vi "HTML Video Steams.vi"(7 "Cameras 2":refnum<vi>, 8 "Exit":refnum<vi>, 10 "Video Feed 2":refnum<vi>, 11 "Automation Refnum in":refnum<k7>) -> (0 "error out":errorcluster, 3 "Automation Refnum out":refnum<k7>)   [LabVIEW 2017]
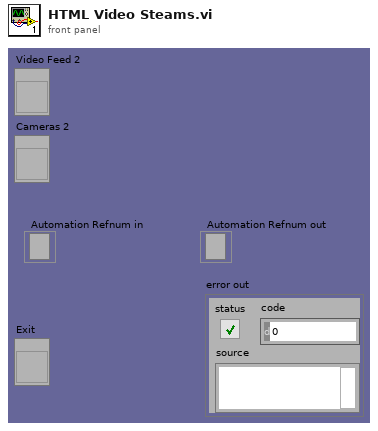
[diagram p1: front panel]
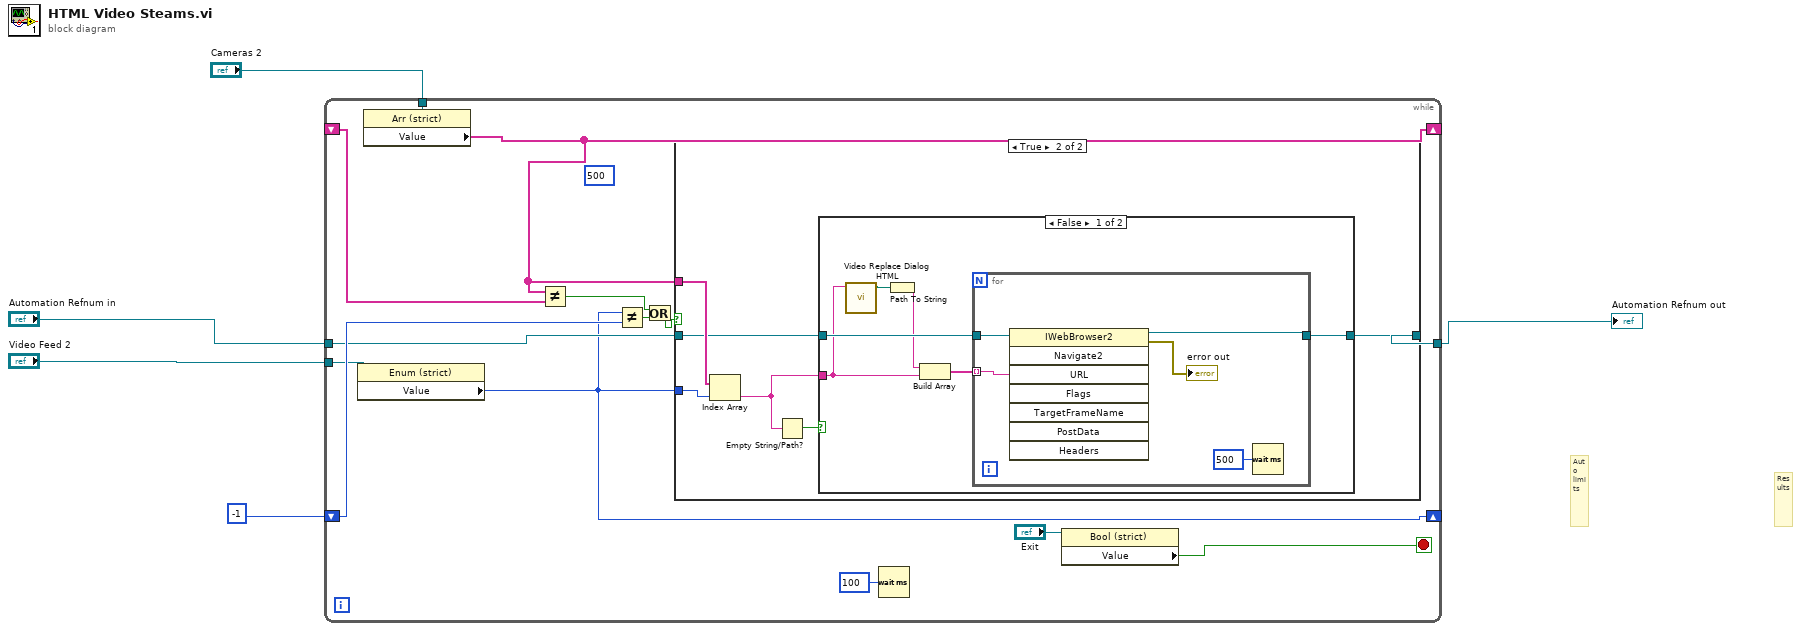
[diagram p0: block diagram]
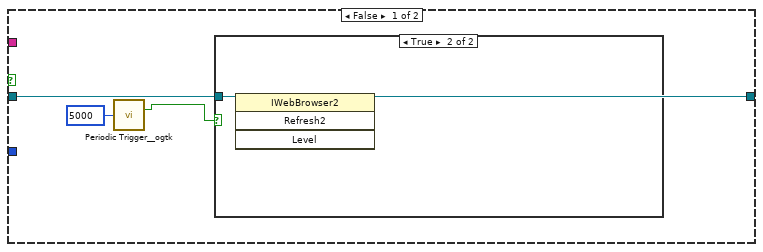
[diagram p2: hidden frame]
diagram:
  # "Results"
  # "Auto limits"
  n1 = while {
    shift-right: [w13] -> _
    shift-left: -1 -> [w18]
    tunnel: "Video Feed 2" -> [w14]
    tunnel: "Automation Refnum in" -> [w17]
    tunnel: [w19] -> w5
    shift-right: [w6] -> _
    shift-left: _ -> [w9]
    tunnel: "Cameras 2" -> [w7]
    stop <- w15 stop-if-true
    (unwired) 500
    n2 = property class="Enum (strict)"(reference=w14) -> ("Value"=w13:enum16{"Camera 1", "Camera2", "Mobile"})  [unwired: 1 in, 2 out]
    n3 = property class="Arr (strict)"(reference=w7) -> ("Value"=w6:string[])  [unwired: 1 in, 2 out]
    n4 = Not Equal?(x=w6, y=w9) -> (x != y?=w8:bool)
    n5 = Not Equal?(x=w13, y=w18) -> (x != y?=w11:bool)
    n6 = Or(x=w8, y=w11) -> (x .or. y?=w10:bool)
    n7 = case shown="True" w10 {
      tunnel: [w22 w29] -> w19
      tunnel: w6 -> [_ w28]
      tunnel: w13 -> [_ w27]
      tunnel: w17 -> [w22 w26]
      frame False {
        n8 = call <userlib>:"Periodic Trigger__ogtk.vi"("time (ms)"=u32 5000) -> ("Triggered"=w21:bool)  [unwired: 12 in, 2 out]
        n9 = case shown="True" w21 {
          tunnel: w22 -> [_ w23]
          frame False {
          }
          frame True {
            n10 = invoke class="IWebBrowser2" method="Refresh2"(reference=w23) -> ()  [unwired: 3 in, 4 out]
          }
        }
      }
      frame True {
        n11 = Index Array(array=w28, index=w27) -> (element=w25:string)
        n12 = Empty String/Path?(string/path=w25) -> (empty?=w24:bool)
        n13 = case shown="False" w24 {
          tunnel: [w35 w41] -> w29
          tunnel: w26 -> [w34 w41]
          tunnel: w25 -> [w31 _]
          frame False {
            n14 = call "Video Replace Dialog HTML.vi"("String"=w31) -> ("appended path"=w30:path)  [unwired: 10 in]
            n15 = Path To String(path=w30) -> (string=w33:string)
            n16 = Build Array(w33, w31) -> (w32:string[])
            n17 = for {
              tunnel: w32 -> [w37] mode=indexing
              tunnel: w34 -> [w38]
              tunnel: [w40] -> w35
              n18 = invoke class="IWebBrowser2" method="Navigate2"(reference=w38, "URL"=w37) -> (reference out=w40:refnum<k7>, error out=→"error out":errorcluster)  [unwired: 6 in, 6 out]
              n19 = Wait (ms)(milliseconds to wait=u32 500) -> ()  [unwired: 1 out]
            }
          }
          frame True {
          }
        }
      }
    }
    n20 = Wait (ms)(milliseconds to wait=u32 100) -> ()  [unwired: 1 out]
    n21 = property class="Bool (strict)"(reference="Exit") -> ("Value"=w15:bool)  [unwired: 1 in, 2 out]
  }
  "Automation Refnum out" <- w5
